vi "welcome.vi"(4 "error in":errorcluster, 7 "Version":string) -> (0 "error out":errorcluster)   [LabVIEW 2016]
uses:
  <vilib>/Utility/miscctls.llb/LVPointTypeDef.ctl
panel:
  out "eye":bool
  # "Animal Training"
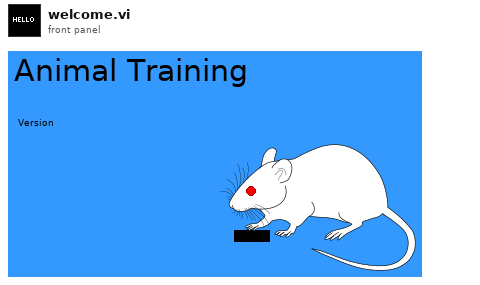
[diagram p1: front panel]
types:
  T1 = typedef "LVPointTypeDef.ctl" = cluster{"Horizontal":i16, "Vertical":i16}
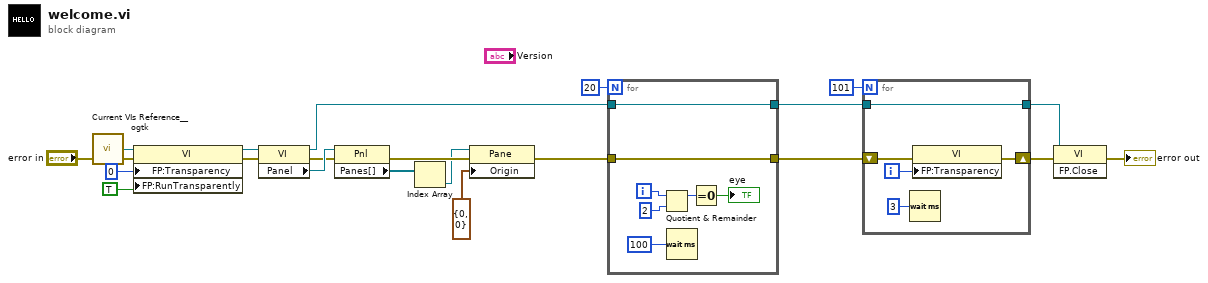
[diagram p0: block diagram]
diagram:
  n1 = call <userlib>:"Current VIs Reference__ogtk.vi"() -> ("Current VI's reference"=w15:refnum<vi>)  [unwired: 5 in]
  n2 = property class="VI"(reference=w15, error in="error in", "FP:Transparency"=u8 0 ("Front Panel Window:Transparency"), "FP:RunTransparently"=TRUE ("Front Panel Window:Run VI Transparently")) -> (reference out=w14:refnum<vi>, error out=w13:errorcluster)
  n3 = property class="VI"(reference=w14, error in=w13) -> (reference out=w1:refnum<vi>, error out=w16:errorcluster, "Panel"=w21:refnum<vi>)
  n4 = property class="Pnl"(reference=w21, error in=w16) -> (error out=w19:errorcluster, "Panes[]"=w17:refnum<vi>[])  [unwired: 1 out]
  n5 = Index Array(array=w17) -> (element=w18:refnum<vi>)  [unwired: 1 in]
  n6 = property class="Pane"(reference=w18, error in=w19, "Origin"=T1 {"Horizontal"=0, "Vertical"=0}) -> (error out=w3:errorcluster)  [unwired: 1 out]
  n7 = for {
    N: 20 -> [_]
    tunnel: w3 -> [w23]
    tunnel: [w23] -> w2
    tunnel: [w22] -> w7
    tunnel: w1 -> [w22]
    i -> [w28]
    n8 = Quotient & Remainder(x=w28, y=2) -> (x-y*floor(x/y)=w26:i32)  [unwired: 1 out]
    n9 = Wait (ms)(milliseconds to wait=u32 100) -> ()  [unwired: 1 out]
    n10 = Equal To 0?(x=w26) -> (x = 0?=→"eye":bool)
  }
  n11 = for {
    N: 101 -> [_]
    shift-right: [w31] -> w4
    shift-left: w2 -> [w32]
    tunnel: w7 -> [w33]
    tunnel: [w33] -> w9
    i -> [w30]
    n12 = Wait (ms)(milliseconds to wait=u32 3) -> ()  [unwired: 1 out]
    n13 = property class="VI"(error in=w32, "FP:Transparency"=w30) -> (error out=w31:errorcluster)  [unwired: 1 in, 1 out]
  }
  n14 = invoke class="VI" method="FP.Close"(reference=w9, error in=w4) -> (error out=→"error out":errorcluster)  [unwired: 1 in, 2 out]
